vi "FormulaAddIO.vi"(0 "__args":T1) -> (2 "__errStatus":bool, 3 "__errCode":i32, 4 "__errSource":string)   [LabVIEW 2013]
panel:
  out "__return":cluster{"UID":i32, "UID":i32}
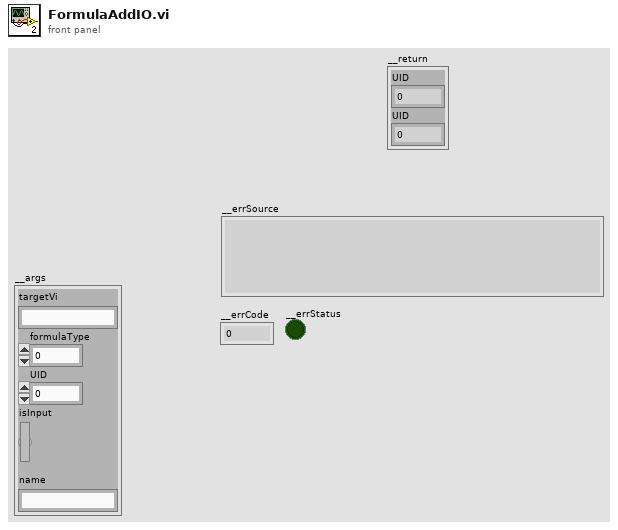
[diagram p1: front panel]
types:
  T1 = cluster{"targetVi":string, "formulaType":i32, "UID":i32, "isInput":bool, "name":string}
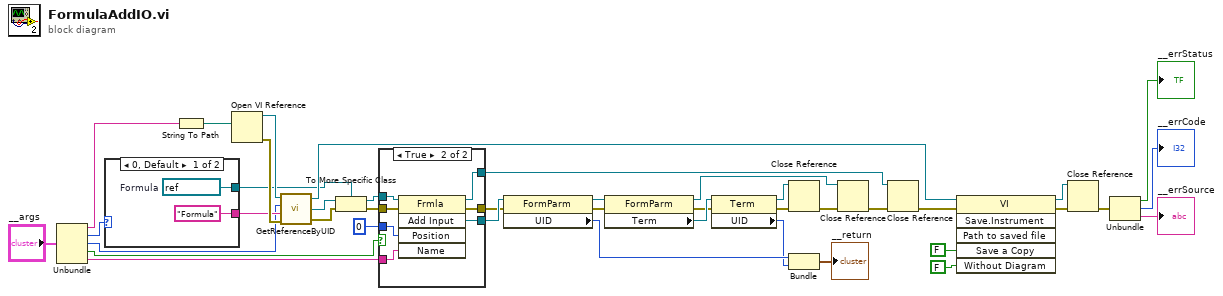
[diagram p0: block diagram]
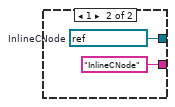
[diagram p2: hidden frame]
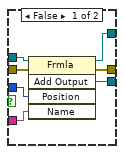
[diagram p3: hidden frame]
diagram:
  n1 = Unbundle("__args") -> ("targetVi"=w35:string, "formulaType"=w8:i32, "UID"=w9:i32, "isInput"=w11:bool, "name"=w10:string)
  n2 = case shown="0, Default" w8 {
    tunnel: [w43 w45] -> w13
    tunnel: ["Formula" ("objectClass") "InlineCNode" ("objectClass")] -> w12
    frame 0, Default {
      w43 = refnum<vi> refnum  # Formula
    }
    frame 1 {
      w45 = refnum<vi> refnum  # InlineCNode
    }
  }
  n3 = String To Path(string=w35) -> (path=w37:path)
  n4 = Open VI Reference(vi path=w37) -> (vi reference=w34:refnum<vi>, error out=w36:errorcluster)  [unwired: 5 in]
  n5 = call "GetReferenceByUID.vi"("error in (no error)"=w36, "objectClass"=w12, "UID"=w9, "targetVI"=w34) -> ("error out"=w33:errorcluster, "refNum"=w32:refnum<vi>, "dup targetVI"=w17:refnum<vi>)
  n6 = To More Specific Class(target class=w13, reference=w32, error in=w33) -> (specific class reference=w31:refnum<vi>, error out=w30:errorcluster)
  n7 = case shown="True" w11 {
    tunnel: w31 -> [w52 w59]
    tunnel: w30 -> [w51 w58]
    tunnel: [w50 w57] -> w29
    tunnel: [w48 w56] -> w7
    tunnel: [w49 w55] -> w5
    tunnel: u32 0 ("Position") -> [w47 w54]
    tunnel: w10 -> [w46 w53]
    frame False {
      n8 = invoke class="Frmla" method="Add Output"(reference=w52, error in=w51, "Position"=w47, "Name"=w46) -> (reference out=w50:refnum<vi>, error out=w49:errorcluster, "Add Output"=w48:refnum<vi>)  [unwired: 1 in, 2 out]
    }
    frame True {
      n9 = invoke class="Frmla" method="Add Input"(reference=w59, error in=w58, "Position"=w54, "Name"=w53) -> (reference out=w57:refnum<vi>, error out=w55:errorcluster, "Add Input"=w56:refnum<vi>)  [unwired: 1 in, 2 out]
    }
  }
  n10 = property class="FormParm"(reference=w7, error in=w5) -> (reference out=w6:refnum<vi>, error out=w4:errorcluster, "UID"=w3:i32)
  n11 = property class="FormParm"(reference=w6, error in=w4) -> (reference out=w20:refnum<vi>, error out=w25:errorcluster, "Term"=w26:refnum<vi>)
  n12 = property class="Term"(reference=w26, error in=w25) -> (reference out=w21:refnum<vi>, error out=w22:errorcluster, "UID"=w2:i32)
  n13 = Close Reference(reference=w21, error in (no error)=w22) -> (error out=w24:errorcluster)
  n14 = Bundle("UID"=w3, "UID"=w2) -> (→"__return":cluster{"UID":i32, "UID":i32})  [unwired: 1 in]
  n15 = Close Reference(reference=w20, error in (no error)=w24) -> (error out=w23:errorcluster)
  n16 = Close Reference(reference=w29, error in (no error)=w23) -> (error out=w16:errorcluster)
  n17 = invoke class="VI" method="Save.Instrument"(reference=w17, error in=w16, "Save a Copy"=FALSE, "Without Diagram"=FALSE) -> (reference out=w14:refnum<vi>, error out=w15:errorcluster)  [unwired: 2 in, 4 out]
  n18 = Close Reference(reference=w14, error in (no error)=w15) -> (error out=w28:errorcluster)
  n19 = Unbundle(w28) -> ("status"=→"__errStatus":bool, "code"=→"__errCode":i32, "source"=→"__errSource":string)
